vi "Forces (SubVI).vi"(1 "Data":dbl[][](array[numeric]), 3 "act_b":dbl[](array[numeric]), 5 "Pdin [Pa], Patm [Pa], Temp [K], airflow velocity [m/s]":T8, 7 "AoA_pitch [rad], AoA_yaw [rad], Stream direction [rad]":T5, 9 "Vehicle Parameters":T2, 11 "Fe_data":dbl[](array[numeric]), 12 "i, sim_running, t[s], dt[s]":T3, 13 "V(i) [m/s] NWU, latd(i) [rad], lon(i) [rad], height(i) [m]":T7, 14 "Rotation":T1) -> (4 "M_alpha [rad/s^2], M_beta [rad/s^2]":T4, 6 "acc [m/s^2]":dbl[](array[numeric]), 10 "FE_b [N], FG [N], FA [N], Fco[N]":T6, 15 "FE [N]":dbl[](array[numeric]))   [LabVIEW 2017]
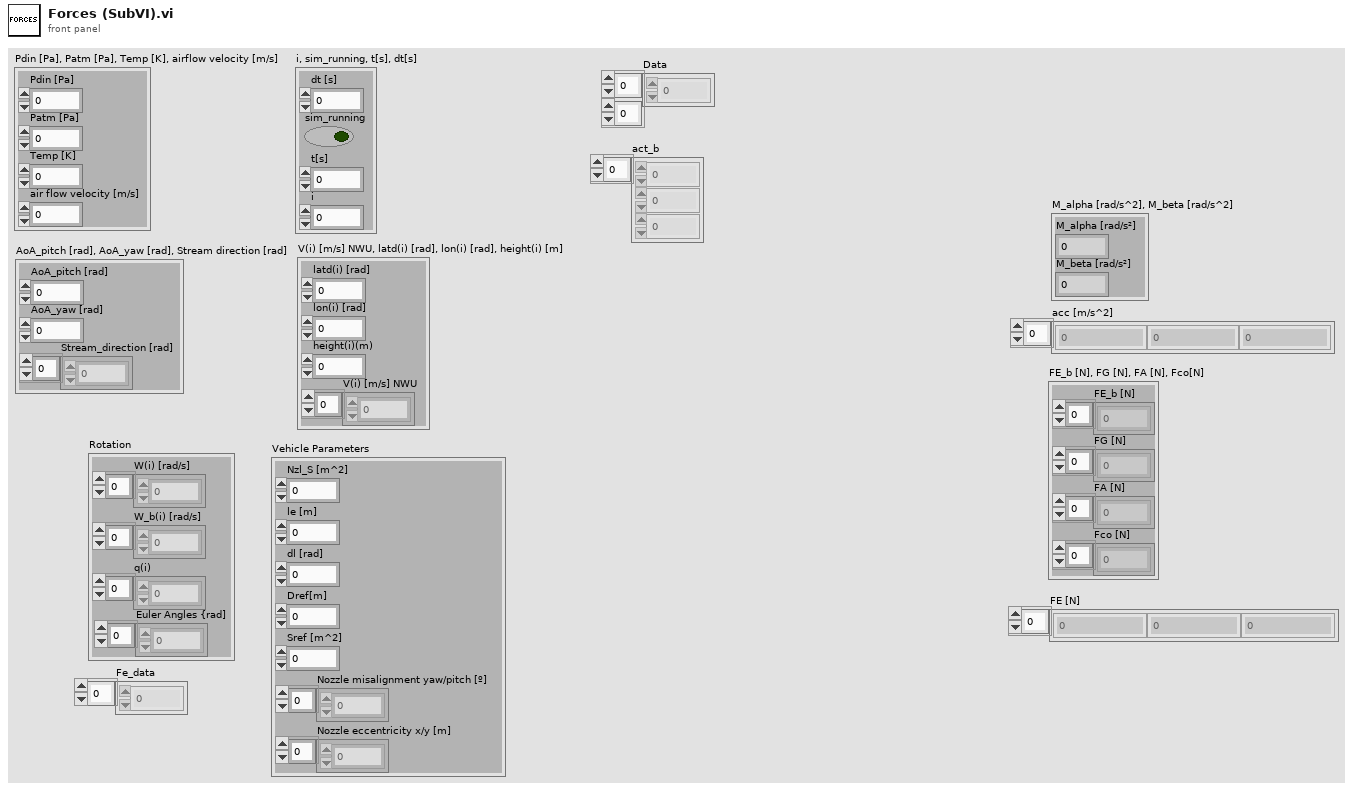
[diagram p1: front panel]
types:
  T1 = cluster{"W(i) [rad/s]":dbl[], "W_b(i) [rad/s]":dbl[], "q(i)":dbl[], "Euler Angles {rad]":dbl[]}
  T2 = cluster{"Nzl_S [m^2]":dbl, "le [m]":dbl, "dl [rad]":dbl, "Dref[m]":dbl, "Sref [m^2]":dbl, "Nozzle misalignment yaw/pitch [º]":dbl[], "Nozzle eccentricity x/y [m]":dbl[]}
  T3 = cluster{"dt [s]":dbl, "sim_running":bool, "t[s]":dbl, "i":i32}
  T4 = cluster{"M_alpha [rad/s²]":dbl, "M_beta [rad/s²]":dbl}
  T5 = cluster{"AoA_pitch [rad]":dbl, "AoA_yaw [rad]":dbl, "Stream_direction [rad]":dbl[]}
  T6 = cluster{"FE_b [N]":dbl[], "FG [N]":dbl[], "FA [N]":dbl[], "Fco [N]":dbl[]}
  T7 = cluster{"latd(i) [rad]":dbl, "lon(i) [rad]":dbl, "height(i)(m)":dbl, "V(i) [m/s] NWU":dbl[]}
  T8 = cluster{"Pdin [Pa]":dbl, "Patm [Pa]":dbl, "Temp [K]":dbl, "air flow velocity [m/s]":dbl}
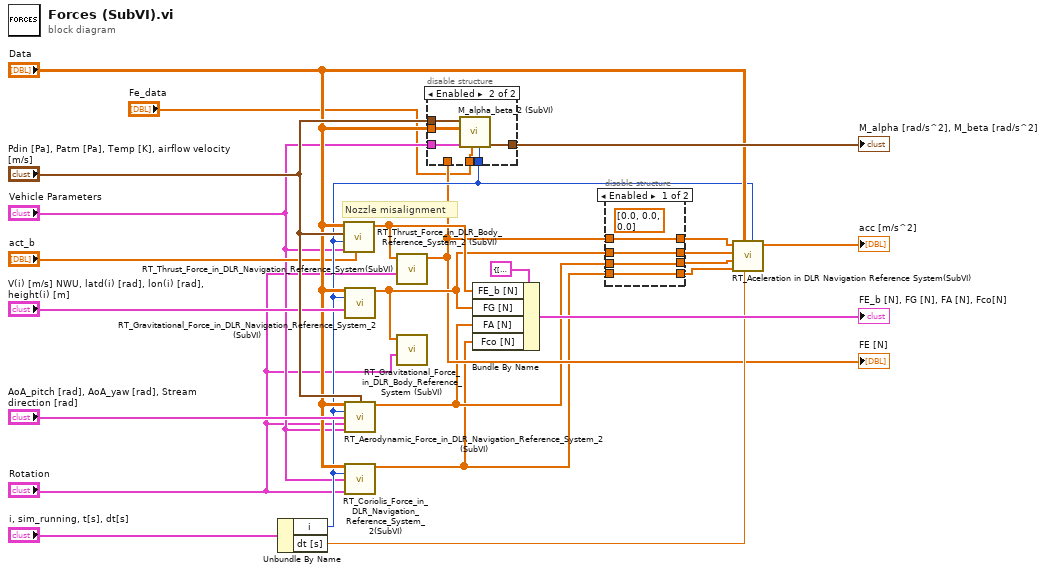
[diagram p0: block diagram]
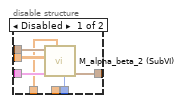
[diagram p2: hidden frame]
diagram:
  # "Nozzle misalignment"
  n1 = Unbundle By Name("i, sim_running, t[s], dt[s]") -> ("i"=w14:i32, "dt [s]"=w21:dbl)
  n2 = call "RT_Thrust_Force_in_DLR_Body_Reference_System_2 (SubVI).vi"("Act_b(i)"="act_b", "Vehicle Parameters"="Vehicle Parameters", "i"=w14, "cluster"="Pdin [Pa], Patm [Pa], Temp [K], airflow velocity [m/s]", "Data"="Data") -> ("FE_b"=w15:dbl[])  [unwired: 6 in]
  n3 = call "RT_Gravitational_Force_in_DLR_Navigation_Reference_System_2 (SubVI).vi"("Data"="Data", "i"=w14, "input cluster"="V(i) [m/s] NWU, latd(i) [rad], lon(i) [rad], height(i) [m]") -> ("FG_d"=w9:dbl[])  [unwired: 11 in, 1 out]
  n4 = call "RT_Aerodynamic_Force_in_DLR_Navigation_Reference_System_2 (SubVI).vi"("Data"="Data", "input cluster 3"="Pdin [Pa], Patm [Pa], Temp [K], airflow velocity [m/s]", "i"=w14, "output cluster"="AoA_pitch [rad], AoA_yaw [rad], Stream direction [rad]", "Rotation"="Rotation", "Vehicle Parameters"="Vehicle Parameters") -> ("FA"=w5:dbl[])  [unwired: 8 in, 1 out]
  n5 = call "RT_Coriolis_Force_in_DLR_Navigation_Reference_System_2(SubVI).vi"("Data"="Data", "i"=w14, "Vehicle Parameters"="Vehicle Parameters", "Rotation"="Rotation") -> ("Fco (N)"=w3:dbl[])  [unwired: 11 in]
  n6 = call "RT_Thrust_Force_in_DLR_Navigation_Reference_System(SubVI).vi"("Rotation"="Rotation", "FE_b"=w15) -> ("FE"=w7:dbl[])  [unwired: 8 in]
  "FE [N]" <- w7
  n7 = call "RT_Gravitational_Force_in_DLR_Body_Reference_System (SubVI).vi"("Rotation"="Rotation", "FG_d"=w9) -> ()  [unwired: 9 in, 1 out]
  n8 = disable-structure shown="Enabled" {
    disable-tunnel: "Pdin [Pa], Patm [Pa], Temp [K], airflow velocity [m/s]" -> [w30 w36]
    disable-tunnel: [w29 w32] -> w19
    disable-tunnel: "Data" -> [w28 w33]
    disable-tunnel: w14 -> [w27 w35]
    disable-tunnel: "Vehicle Parameters" -> [w26 w34]
    disable-tunnel: w7 -> [w25 _]
    disable-tunnel: "Fe_data" -> [_ w31]
    frame Disabled {
      n9 = call "M_alpha_beta_2 (SubVI).vi"("i"=w27, "FE [N]"=w25, "Vehicle Parameters"=w26, "Data"=w28, "cluster"=w30) -> ("output cluster"=w29:T4)  [unwired: 4 in, 2 out]
    }
    frame Enabled {
      n10 = call "M_alpha_beta_2 (SubVI).vi"("i"=w35, "Fe_data"=w31, "Vehicle Parameters"=w34, "Data"=w33, "cluster"=w36) -> ("output cluster"=w32:T4)  [unwired: 4 in, 2 out]
    }
  }
  "M_alpha [rad/s^2], M_beta [rad/s^2]" <- w19
  n11 = Bundle By Name(cluster=T6 {"FE_b [N]"=[], "FG [N]"=[], "FA [N]"=[], "Fco [N]"=[]} ("output cluster 2"), "FE_b [N]"=w15, "FG [N]"=w9, "FA [N]"=w5, "Fco [N]"=w3) -> (→"FE_b [N], FG [N], FA [N], Fco[N]":T6)
  n12 = disable-structure shown="Enabled" {
    disable-tunnel: w9 -> [w39 w44]
    disable-tunnel: [w39 w44] -> w8
    disable-tunnel: w7 -> [w38 w43]
    disable-tunnel: [w38 w43] -> w6
    disable-tunnel: w5 -> [w37 w42]
    disable-tunnel: [w37 w42] -> w4
    disable-tunnel: w3 -> [w40 w41]
    disable-tunnel: [w40 w41] -> w2
    frame Enabled {
      (unwired) dbl[] [0.0, 0.0, 0.0] ("FG_d")
    }
    frame Disabled {
    }
  }
  n13 = call "RT_Aceleration in DLR Navigation Reference System(SubVI).vi"("i"=w14, "dt(s)"=w21, "Data"="Data", "Fco (N)"=w2, "FA"=w4, "FG"=w8, "FE"=w6) -> ("acc"=→"acc [m/s^2]":dbl[])  [unwired: 4 in]
